vi "ShooterTest.vi"() -> ()   [LabVIEW 2013]
uses:
  <vilib>/Rock Robotics/SystemInterfaces/Typedef/FPGA_TypedefSolenoidModule.ctl
  <vilib>/Rock Robotics/WPI/Solenoid/WPI_SolenoidChannel.ctl
  Robot_Framework_2014/SingleSolenoidAction.ctl
  <vilib>/Rock Robotics/WPI/Joystick/WPI_JoystickDeviceEnum.ctl
  <vilib>/Rock Robotics/SystemInterfaces/DIO/FPGA_DIOChannel.ctl
  <vilib>/Rock Robotics/SystemInterfaces/Typedef/FPGA_TypedefDigitalModule.ctl
  <vilib>/Rock Robotics/SystemInterfaces/DIO/FPGA_DIORelayChannel.ctl
  <vilib>/Rock Robotics/WPI/Solenoid/WPI_SolenoidOpenSingle.vi
panel:
  in  "Kicker Module":T1
  in  "Kicker Channel":T2
  in  "Firing Channel":T2
  in  "Firing Module":T1
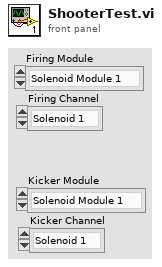
[diagram p1: front panel]
types:
  T1 = typedef "FPGA_TypedefSolenoidModule.ctl" = enum16{"Solenoid Module 1", "Solenoid Module 2"}
  T2 = typedef "WPI_SolenoidChannel.ctl" = enum8{"Solenoid 1", "Solenoid 2", "Solenoid 3", "Solenoid 4", "Solenoid 5", "Solenoid 6", "Solenoid 7", "Solenoid 8", "Invalid"}
  T3 = typedef "FPGA_DIORelayChannel.ctl" = enum8{"Relay 1", "Relay 2", "Relay 3", "Relay 4", "Relay 5", "Relay 6", "Relay 7", "Relay 8", "Invalid"}
  T4 = typedef "FPGA_TypedefDigitalModule.ctl" = enum16{"Digital Module 1", "Digital Module 2"}
  T5 = typedef "FPGA_DIOChannel.ctl" = enum8{"DIO 1", "DIO 2", "DIO 3", "DIO 4", "DIO 5", "DIO 6", "DIO 7", "DIO 8", "DIO 9", "DIO 10", "DIO 11", "DIO 12", "DIO 13", "DIO 14", "Invalid"}
  T6 = typedef "WPI_JoystickDeviceEnum.ctl" = enum16{"USB 1", "USB 2", "USB 3", "USB 4", "Kinect 1", "Kinect 2"}
  T7 = typedef "SingleSolenoidAction.ctl" = enum16{"Init", "SetState", "Disable"}
  T8 = typedef "WPI_JoystickDevRef.ctl" = cluster{"Device":T6}
  T9 = typedef "WPI_SolenoidDevRef.ctl" = cluster{"DevStatus":errorcluster, "Solenoid Module":T1, "Forward Solenoid Channel":T2, "Reverse Solenoid Channel":T2}
  T10 = typedef "WPI_CompressorDevRef.ctl" = cluster{"DevStatus":errorcluster, "DigitalInputDevRef":T11, "RelayDevRef":T12}
  T11 = typedef "WPI_DigitalInputDevRef.ctl" = cluster{"DevStatus":errorcluster, "DIO Channel":T5, "Digital Module":T4}
  T12 = typedef "WPI_RelayDevRef.ctl" = cluster{"DevStatus":errorcluster, "Relay Channel":T3, "Digital Module":T4, "Relay Direction":T13}
  T13 = typedef "WPI_RelayDirection.ctl" = enum16{"Both directions", "Forward only", "Reverse only"}
  T14 = typedef "WPI_JoystickButtonState.ctl" = cluster{"Button 1":bool, "Button 2":bool, "Button 3":bool, "Button 4":bool, "Button 5":bool, "Button 6":bool, "Button 7":bool, "Button 8":bool, "Button 9":bool, "Button 10":bool, "Button 11":bool, "Button 12":bool}
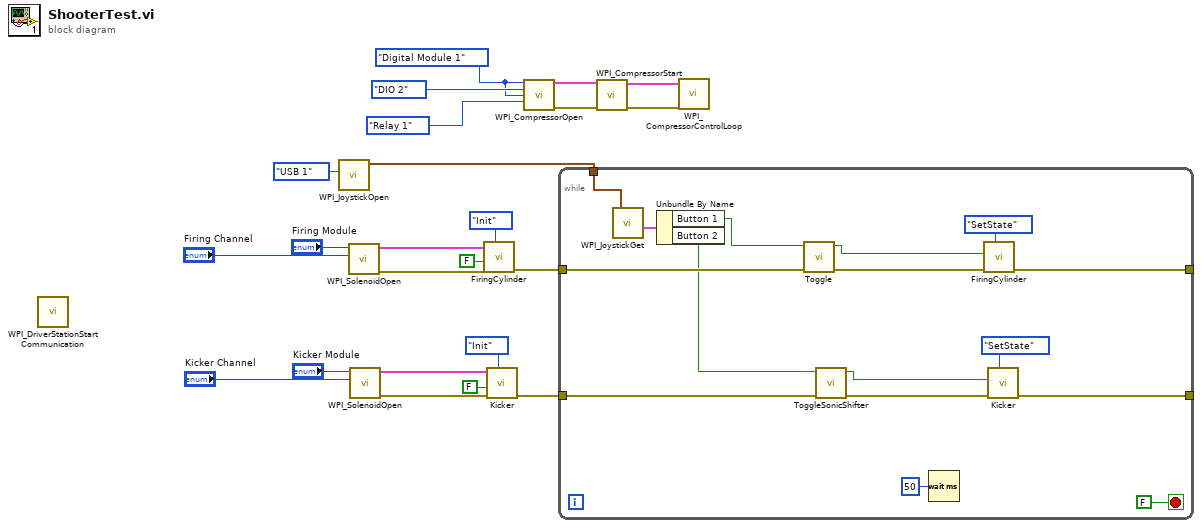
[diagram p0: block diagram]
diagram:
  w6 = FPGA_TypedefDigitalModule."Digital Module 1" ("Pressure Switch Digital Module (Module 1)")
  n1 = call <vilib>:"WPI_DriverStationStart Communication.vi"() -> ()  [unwired: 12 in]
  n2 = call <vilib>:"WPI_JoystickOpen.vi"("JoystickDevice"=WPI_JoystickDeviceEnum."USB 1") -> ("JoystickDevRef"=w9:T8)  [unwired: 10 in]
  n3 = call-poly <vilib>:"WPI_SolenoidOpen.vi"("Solenoid Channel"="Firing Channel", "Solenoid Module (Module 1)"="Firing Module") -> ("error out"=w11:errorcluster, "SolenoidDevRef"=w12:T9)  [unwired: 8 in]
  n4 = call-poly <vilib>:"WPI_SolenoidOpen.vi"("Solenoid Channel"="Kicker Channel", "Solenoid Module (Module 1)"="Kicker Module") -> ("error out"=w10:errorcluster, "SolenoidDevRef"=w13:T9)  [unwired: 8 in]
  n5 = call "FiringCylinder.vi"("Action"=SingleSolenoidAction."Init", "error in (no error)"=w11, "Default Position"=FALSE, "SolenoidDevRef"=w12) -> ("error out"=w21:errorcluster)  [unwired: 7 in]
  n6 = call "Kicker.vi"("Action"=SingleSolenoidAction."Init", "error in (no error)"=w10, "Default Position"=FALSE, "SolenoidDevRef"=w13) -> ("error out"=w20:errorcluster)  [unwired: 7 in]
  n7 = call <vilib>:"WPI_CompressorOpen.vi"("Pressure Switch Digital Module (Module 1)"=w6, "Pressure Switch DIO Channel"=FPGA_DIOChannel."DIO 2", "Relay Digital Module (Module 1)"=w6, "Relay Channel"=FPGA_DIORelayChannel."Relay 1") -> ("CompressorDevRef"=w4:T10, "error out"=w2:errorcluster)  [unwired: 10 in]
  n8 = while {
    tunnel: [w35] -> _
    tunnel: [w34] -> _
    tunnel: w21 -> [w33]
    tunnel: w20 -> [w32]
    tunnel: w9 -> [w31]
    stop <- FALSE stop-if-true
    n9 = call <vilib>:"WPI_JoystickGet.vi"("JoystickDevRef"=w31) -> ("Buttons"=w29:T14)  [unwired: 4 in, 2 out]
    n10 = Unbundle By Name(w29) -> ("Button 1"=w28:bool, "Button 2"=w26:bool)
    n11 = call "Toggle.vi"("error in"=w33, "RawInput"=w28) -> ("error out"=w30:errorcluster, "ToggleState"=w24:bool)  [unwired: 8 in]
    n12 = call "ToggleSonicShifter.vi"("error in"=w32, "cSonicShifter"=w26) -> ("error out"=w27:errorcluster, "Actuate?"=w25:bool)  [unwired: 8 in]
    n13 = Wait (ms)(milliseconds to wait=u32 50) -> ()  [unwired: 1 out]
    n14 = call "FiringCylinder.vi"("Action"=SingleSolenoidAction."SetState", "error in (no error)"=w30, "Actuate?"=w24) -> ("error out"=w34:errorcluster)  [unwired: 8 in]
    n15 = call "Kicker.vi"("Action"=SingleSolenoidAction."SetState", "error in (no error)"=w27, "Actuate?"=w25) -> ("error out"=w35:errorcluster)  [unwired: 8 in]
  }
  n16 = call <vilib>:"WPI_CompressorStart.vi"("error in (no error)"=w2, "CompressorDevRef"=w4) -> ("error out"=w1:errorcluster, "CompressorDevRef"=w3:T10)  [unwired: 8 in]
  n17 = call <vilib>:"WPI_CompressorControlLoop.vi"("error in (no error)"=w1, "CompressorDevRef"=w3) -> ()  [unwired: 10 in]
